vi "deneme.vi"() -> ()   [LabVIEW 2019]
uses:
  <vilib>/Utility/file.llb/Read Delimited Spreadsheet (DBL).vi
panel:
  out "Rem Mag":dbl
  out "Slope at coercive field":dbl
  out "Done":bool
  out "Saturation Field":dbl
  out "all rows":dbl[][](array[numeric])
  in  "file path (dialog if empty)":path
  out "Area Enclosed by Hysteresis":dbl
  out "Hn Downwards":dbl
  out "Hn Upwards":dbl
  out "Switching field distribution":dbl
  out "Rigid field offset":dbl
  out "Gradient near H=0":dbl
  out "Initial slope":i32
  out "Saturation field":dbl
  out "Squarness":dbl
  out "Rigid Field":dbl
  out "Coercive field":dbl
  out "Downward":dbl
  out "Upward":dbl
  out "XY Graph":cluster{"data":dbl[], "data":dbl[]}(graph)
  out "subarray asc/desc":dbl[](array[numeric])
  out "subarray y axis":dbl[](array[numeric])
  out "subarray x axis":dbl[](array[numeric])
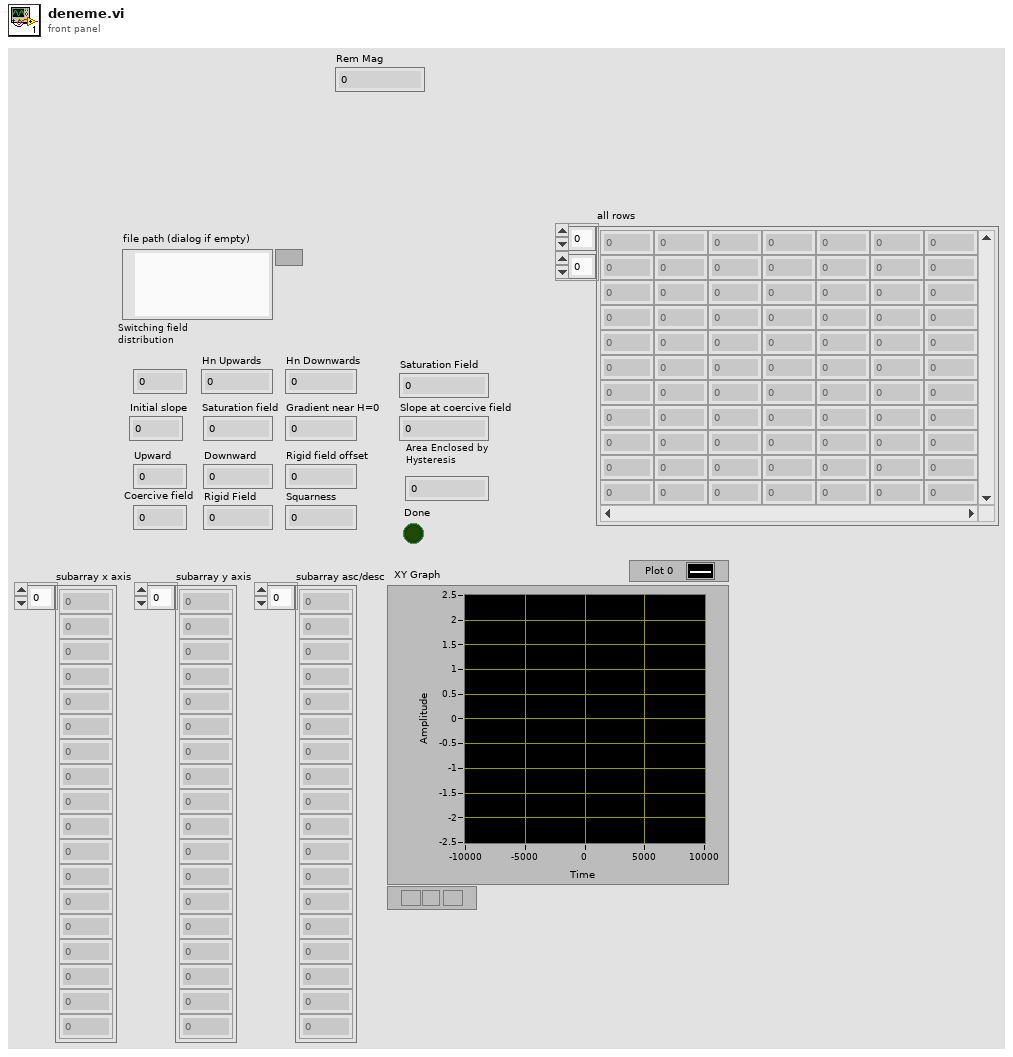
[diagram p1: front panel]
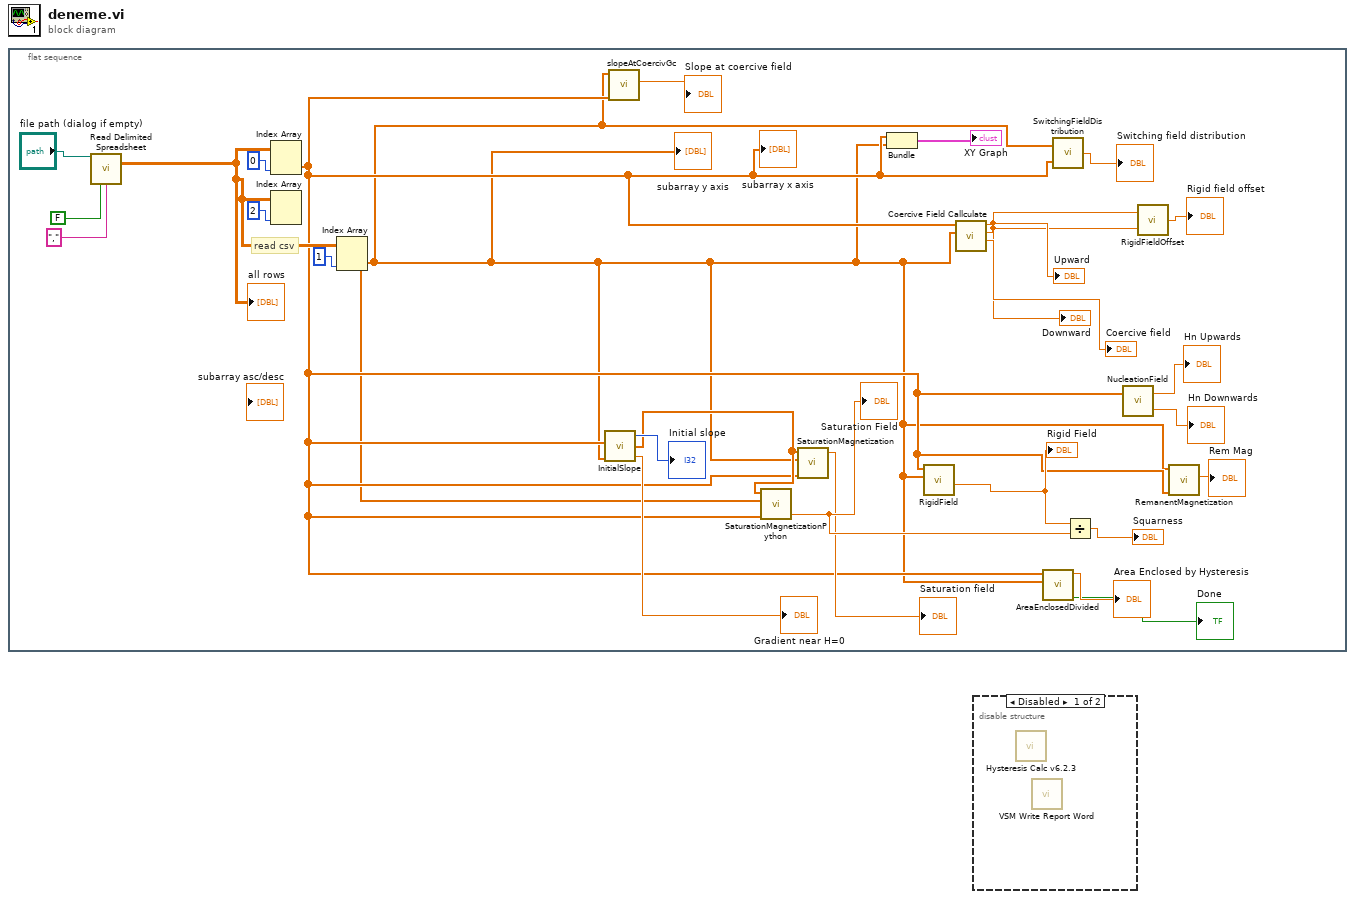
[diagram p0: block diagram]
diagram:
  n1 = flat-sequence {
    frame #0 {
      # "read csv"
      n2 = call-poly <vilib>:"Read Delimited Spreadsheet.vi"("file path (dialog if empty)"="file path (dialog if empty)", "transpose? (F)"=FALSE, "delimiter (\\t)"="," ("delimiter (\\t)")) -> ("all rows"=w6:dbl[][])  [unwired: 7 in, 5 out]
      "all rows" <- w6
      n3 = Index Array(array=w6, index (col)=0 ("disabled index (col)")) -> (element=w3:dbl[])  [unwired: 1 in]
      "subarray x axis" <- w3
      n4 = Index Array(array=w6, index (col)=2 ("disabled index (col)")) -> ()  [unwired: 1 in, 1 out]
      n5 = Index Array(array=w6, index (col)=1 ("disabled index (col)")) -> (element=w2:dbl[])  [unwired: 1 in]
      "subarray y axis" <- w2
      n6 = call "InitialSlope.vi"("H (x-axis)"=w2, "B (y-axis)"=w3) -> ("Initial Slope"=→"Gradient near H=0":dbl, "all gradients"=w12:dbl[], "Index of value closest to 0"=→"Initial slope":i32)  [unwired: 2 in]
      n7 = call "slopeAtCoercivGc.vi"("B"=w3, "H"=w2) -> ("Gc"=→"Slope at coercive field":dbl)  [unwired: 9 in]
      n8 = call "SaturationMagnetizationPython.vi"("B"=w3, "H"=w2, "all gradients"=w12) -> ("Saturation Field"=w9:dbl)  [unwired: 3 in]
      "Saturation Field" <- w9
      n9 = call "SaturationMagnetization.vi"("B"=w3, "H"=w2, "all gradients"=w12) -> ("SaturationField"=→"Saturation field":dbl)  [unwired: 3 in]
      n10 = Bundle("all rows"=w3, "all rows"=w2) -> (→"XY Graph":cluster{"all rows":dbl[], "all rows":dbl[]})  [unwired: 1 in]
      n11 = call "RigidField.vi"("H"=w2, "B"=w3) -> ("Br"=w4:dbl)  [unwired: 7 in, 2 out]
      "Rigid Field" <- w4
      n12 = call "Coercive Field Callculate.vi"("H"=w2, "B"=w3) -> ("Hc"=→"Coercive field":dbl, "Downward"=w20:dbl, "Upward"=w21:dbl)  [unwired: 7 in]
      "Upward" <- w21
      "Downward" <- w20
      n13 = call "AreaEnclosedDivided.vi"("H"=w2, "B"=w3) -> ("Done"=→"Done":bool, "Area"=→"Area Enclosed by Hysteresis":dbl)  [unwired: 8 in]
      n14 = call "SwitchingFieldDistribution.vi"("B"=w3, "H"=w2) -> ("SFD"=→"Switching field distribution":dbl)
      n15 = Divide(x=w4, y=w9) -> (x/y=→"Squarness":dbl)
      n16 = call "NucleationField.vi"("array"=w3) -> ("Nucleation Field Downwards"=→"Hn Downwards":dbl, "Nucleation Field Upwards"=→"Hn Upwards":dbl)  [unwired: 1 in]
      n17 = call "RigidFieldOffset.vi"("Downward's Hc"=w20, "Upward's Hc"=w21) -> ("Rigid Field offset"=→"Rigid field offset":dbl)
      n18 = call "RemanentMagnetization.vi"("B"=w3, "H"=w2) -> ("Rem Mag"=→"Rem Mag":dbl)  [unwired: 9 in]
    }
  }
  n19 = disable-structure shown="Disabled" {
    frame Disabled {
      n20 = call "Hysteresis Calc v6.2.3.vi"() -> ()  [unwired: 17 in, 3 out]
      n21 = call "VSM Write Report Word.vi"() -> ()  [unwired: 19 in, 1 out]
    }
    frame Enabled {
    }
  }
